vi "HeatTape_SubVI_Final.vi"(0 "Modbus Master in":refnum<class "Modbus Master.lvclass">, 1 "serial master instance":refnum<class "Modbus Master.lvclass">, 2 "Hysterisis (Station 01)":string, 3 "Set Value (Station 01)":string, 4 "error in":errorcluster, 5 "Set Value (Station 02)":string, 6 "Hysterisis (Station 02)":string, 7 "error in (no error)":errorcluster, 8 "Slide Refnum 2":refnum<vi>, 10 "WFChart Refnum":refnum<vi>, 12 "Slide Refnum":refnum<vi>) -> (14 "Modbus master out":refnum<class "Modbus Master.lvclass">, 16 "Numeric":dbl, 18 "String 2":string, 20 "Modbus Master out":refnum<class "Modbus Master.lvclass">, 21 "Boolean":bool, 22 "Cluster":cluster{dbl, dbl, dbl, dbl}, 23 "error out 3":errorcluster, 24 "Numeric 2":dbl, 25 "String":string, 26 "Boolean 2":bool, 27 "error out":errorcluster)   [LabVIEW 2019]
uses:
  <vilib>/NI/Modbus Library/API/Master/Modbus Master.lvclass
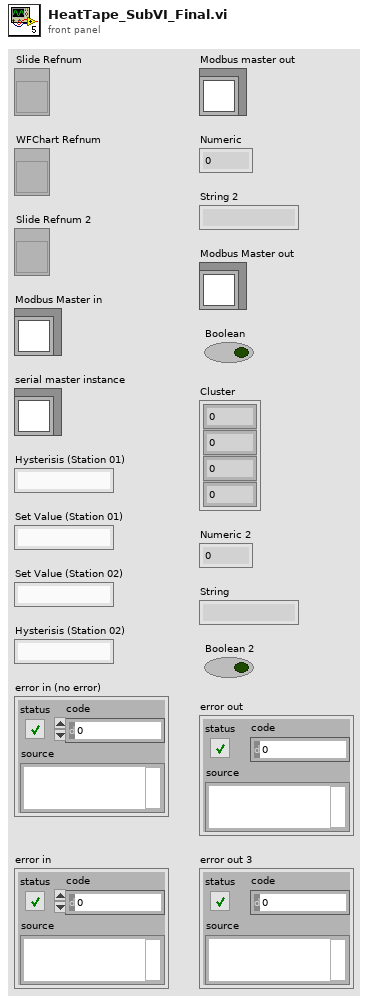
[diagram p1: front panel]
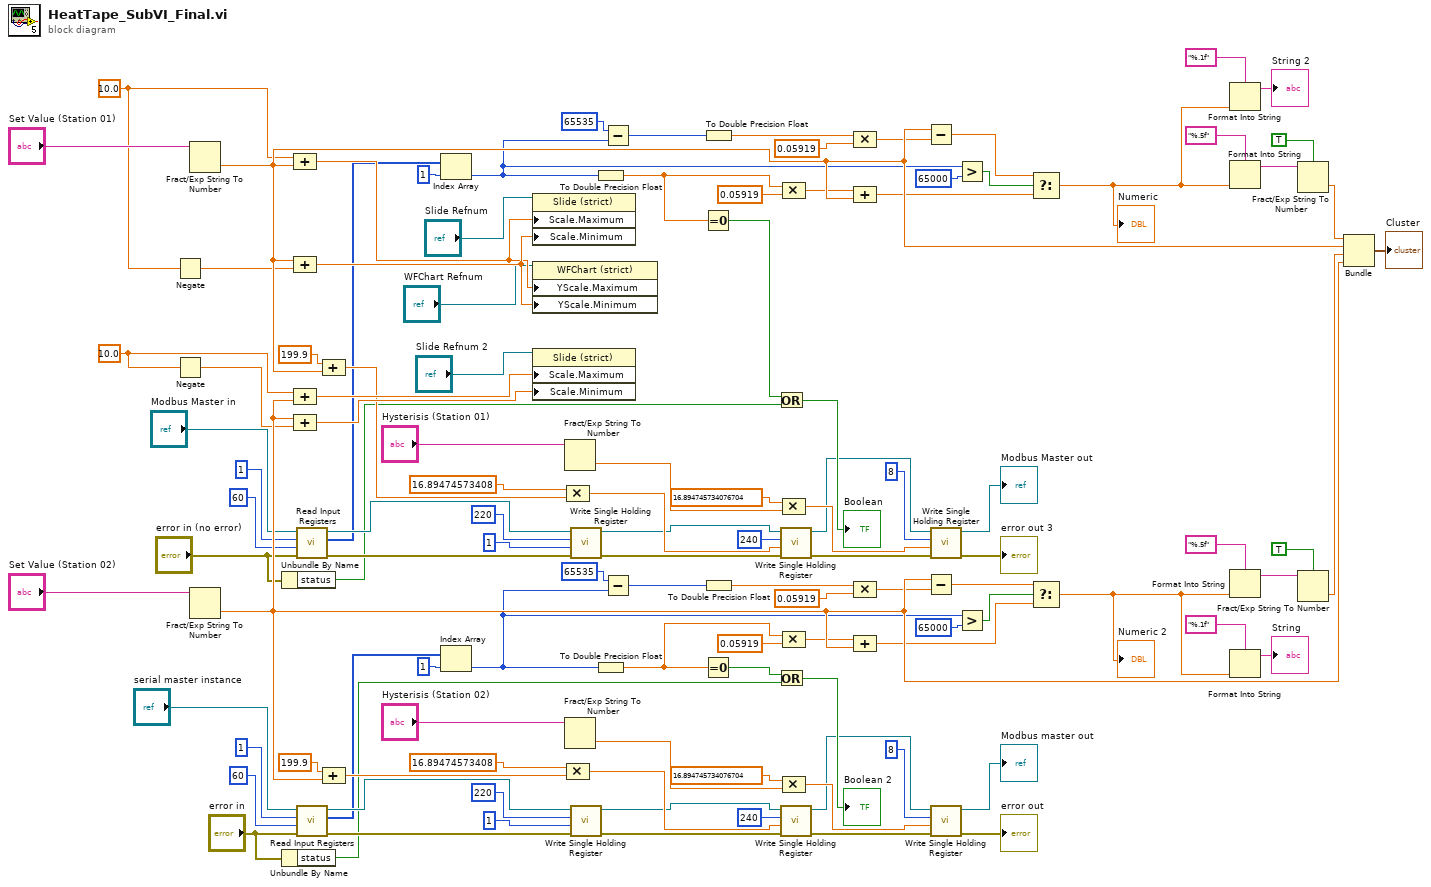
[diagram p0: block diagram]
diagram:
  w73 = 10.0 ("value")
  w26 = 10.0 ("value")
  n1 = Negate(x=w26) -> (-x=w27:dbl)
  n2 = Negate(x=w73) -> (-x=w74:dbl)
  n3 = Fract/Exp String To Number(string="Set Value (Station 01)") -> (number=w42:dbl)  [unwired: 3 in, 1 out]
  n4 = Fract/Exp String To Number(string="Set Value (Station 02)") -> (number=w103:dbl)  [unwired: 3 in, 1 out]
  n5 = Unbundle By Name("error in (no error)") -> ("status"=w16:bool)
  n6 = Unbundle By Name("error in") -> ("status"=w65:bool)
  n7 = Compound Arithmetic op=ADD(w26, w42) -> (w28:dbl)
  n8 = Compound Arithmetic op=ADD(w42, w27) -> (w29:dbl)
  n9 = Compound Arithmetic op=ADD(w73, w103) -> (w75:dbl)
  n10 = Compound Arithmetic op=ADD(w103, w74) -> (w76:dbl)
  n11 = call-dynamic "Read Input Registers.vi"("error in"="error in (no error)", "number of inputs"=u16 60 ("number of inputs (Defaut: 60)"), "starting address"=u16 1 ("starting address (Default: 1)"), "Modbus master in"="Modbus Master in") -> ("error out"=w41:errorcluster, "register values"=w6:u16[], "Modbus master out"=w40:refnum<class "Modbus Master.lvclass">)  [unwired: 5 in]
  n12 = call-dynamic "Read Input Registers.vi"("error in"="error in", "number of inputs"=u16 60 ("number of inputs (Defaut: 60)"), "starting address"=u16 1 ("starting address (Default: 1)"), "Modbus master in"="serial master instance") -> ("error out"=w88:errorcluster, "register values"=w56:u16[], "Modbus master out"=w87:refnum<class "Modbus Master.lvclass">)  [unwired: 5 in]
  n13 = Compound Arithmetic op=ADD(199.9 ("value"), w42) -> (w21:dbl)
  n14 = Compound Arithmetic op=ADD(199.9 ("value"), w103) -> (w68:dbl)
  n15 = Index Array(array=w6, index=1) -> (element=w25:u16)
  n16 = Index Array(array=w56, index=1) -> (element=w72:u16)
  n17 = property on="Property Node" class="Slide (strict)"(reference="Slide Refnum", "Scale.Maximum"=w28, "Scale.Minimum"=w29) -> ()  [unwired: 1 in, 2 out]
  n18 = property on="Property Node" class="WFChart (strict)"(reference="WFChart Refnum", "YScale.Maximum"=w28, "YScale.Minimum"=w29) -> ()  [unwired: 1 in, 2 out]
  n19 = property on="Property Node" class="Slide (strict)"(reference="Slide Refnum 2", "Scale.Maximum"=w75, "Scale.Minimum"=w76) -> ()  [unwired: 1 in, 2 out]
  n20 = Fract/Exp String To Number(string="Hysterisis (Station 01)") -> (number=w51:dbl)  [unwired: 3 in, 1 out]
  n21 = Fract/Exp String To Number(string="Hysterisis (Station 02)") -> (number=w95:dbl)  [unwired: 3 in, 1 out]
  n22 = Compound Arithmetic op=MULTIPLY(16.89474573408 ("value"), w21) -> (w50:dbl)
  n23 = Compound Arithmetic op=MULTIPLY(16.89474573408 ("value"), w68) -> (w94:dbl)
  n24 = call-dynamic "Write Single Holding Register.vi"("error in"=w41, "register to write"=u16 1, "address"=u16 220, "Modbus master in"=w40) -> ("error out"=w47:errorcluster, "Modbus master out"=w46:refnum<class "Modbus Master.lvclass">)  [unwired: 6 in]
  n25 = call-dynamic "Write Single Holding Register.vi"("error in"=w88, "register to write"=u16 1, "address"=u16 220, "Modbus master in"=w87) -> ("error out"=w91:errorcluster, "Modbus master out"=w90:refnum<class "Modbus Master.lvclass">)  [unwired: 6 in]
  n26 = To Double Precision Float(number=w25) -> (double precision float=w15:dbl)
  n27 = To Double Precision Float(number=w72) -> (double precision float=w64:dbl)
  n28 = Subtract(x=u16 65535 ("y"), y=w25) -> (x-y=w32:u16)
  n29 = Subtract(x=u16 65535 ("y"), y=w72) -> (x-y=w79:u16)
  n30 = Equal To 0?(x=w15) -> (x = 0?=w17:bool)
  n31 = Equal To 0?(x=w64) -> (x = 0?=w66:bool)
  n32 = To Double Precision Float(number=w32) -> (double precision float=w30:dbl)
  n33 = To Double Precision Float(number=w79) -> (double precision float=w77:dbl)
  n34 = Or(x=w17, y=w16) -> (x .or. y?=→"Boolean":bool)
  n35 = Or(x=w66, y=w65) -> (x .or. y?=→"Boolean 2":bool)
  n36 = call-dynamic "Write Single Holding Register.vi"("error in"=w47, "register to write"=w50, "address"=u16 240, "Modbus master in"=w46) -> ("error out"=w48:errorcluster, "Modbus master out"=w49:refnum<class "Modbus Master.lvclass">)  [unwired: 6 in]
  n37 = call-dynamic "Write Single Holding Register.vi"("error in"=w91, "register to write"=w94, "address"=u16 240, "Modbus master in"=w90) -> ("error out"=w92:errorcluster, "Modbus master out"=w93:refnum<class "Modbus Master.lvclass">)  [unwired: 6 in]
  n38 = Compound Arithmetic op=MULTIPLY(w15, 0.05919 ("value")) -> (w8:dbl)
  n39 = Compound Arithmetic op=MULTIPLY(16.894745734076704 ("value"), w51) -> (w52:dbl)
  n40 = Compound Arithmetic op=MULTIPLY(w64, 0.05919 ("value")) -> (w58:dbl)
  n41 = Compound Arithmetic op=MULTIPLY(16.894745734076704 ("value"), w95) -> (w96:dbl)
  n42 = Compound Arithmetic op=MULTIPLY(w30, 0.05919 ("value")) -> (w33:dbl)
  n43 = Compound Arithmetic op=ADD(w8, w42) -> (w35:dbl)
  n44 = Compound Arithmetic op=MULTIPLY(w77, 0.05919 ("value")) -> (w80:dbl)
  n45 = Compound Arithmetic op=ADD(w58, w103) -> (w82:dbl)
  n46 = Subtract(x=w42, y=w33) -> (x-y=w34:dbl)
  n47 = Subtract(x=w103, y=w80) -> (x-y=w81:dbl)
  n48 = call-dynamic "Write Single Holding Register.vi"("error in"=w48, "register to write"=w52, "address"=u16 8, "Modbus master in"=w49) -> ("error out"=→"error out 3":errorcluster, "Modbus master out"=→"Modbus Master out":refnum<class "Modbus Master.lvclass">)  [unwired: 6 in]
  n49 = call-dynamic "Write Single Holding Register.vi"("error in"=w92, "register to write"=w96, "address"=u16 8, "Modbus master in"=w93) -> ("error out"=→"error out":errorcluster, "Modbus master out"=→"Modbus master out":refnum<class "Modbus Master.lvclass">)  [unwired: 6 in]
  n50 = Greater?(x=w25, y=u16 65000) -> (0:w36:bool)
  n51 = Greater?(x=w72, y=u16 65000) -> (0:w83:bool)
  n52 = Select(t=w34, s=w36, f=w35) -> (s? t:f=w106:dbl)
  "Numeric" <- w106
  n53 = Select(t=w81, s=w83, f=w82) -> (s? t:f=w105:dbl)
  "Numeric 2" <- w105
  n54 = Format Into String(format string="%.1f", w106) -> (resulting string=→"String 2":string)  [unwired: 2 in, 1 out]
  n55 = Format Into String(format string="%.5f", w106) -> (resulting string=w13:string)  [unwired: 2 in, 1 out]
  n56 = Format Into String(format string="%.5f", w105) -> (resulting string=w63:string)  [unwired: 2 in, 1 out]
  n57 = Format Into String(format string="%.1f", w105) -> (resulting string=→"String":string)  [unwired: 2 in, 1 out]
  n58 = Fract/Exp String To Number(use system decimal point (T)=TRUE, string=w13) -> (number=w18:dbl)  [unwired: 2 in, 1 out]
  n59 = Fract/Exp String To Number(use system decimal point (T)=TRUE, string=w63) -> (number=w102:dbl)  [unwired: 2 in, 1 out]
  n60 = Bundle(w18, w42, w102, w103) -> (→"Cluster":cluster{dbl, dbl, dbl, dbl})  [unwired: 1 in]
